vi "Convolucionador.vi"(9 "df":dbl, 10 "X2":dbl[](array[numeric]), 11 "X1":dbl[](array[numeric])) -> (2 "Areas":dbl[](array[numeric]), 3 "Convolucion":dbl)   [LabVIEW 2017]
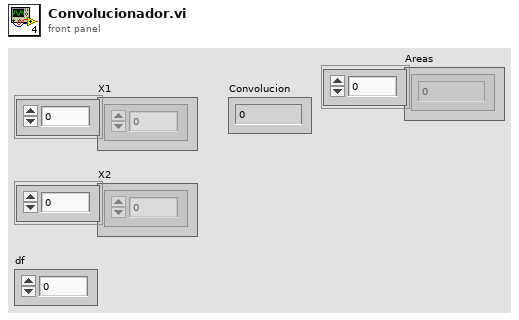
[diagram p1: front panel]
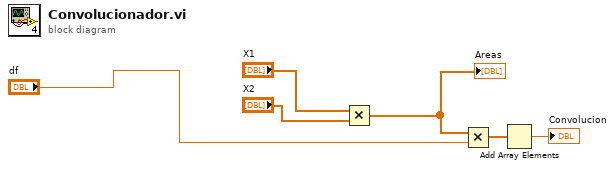
[diagram p0: block diagram]
diagram:
  n1 = Multiply(x="X1", y="X2") -> (x*y=w1:dbl[])
  "Areas" <- w1
  n2 = Multiply(x=w1, y="df") -> (x*y=w6:dbl[])
  n3 = Add Array Elements(numeric array=w6) -> (sum=→"Convolucion":dbl)
